vi "maximini_XYlist_svi.vi"(9 "stored XY":T1, 10 "LY":dbl, 11 "LX":dbl) -> (2 "mini (µm)":dbl, 3 "maxi (µm)":dbl)   [LabVIEW 2013]
uses:
  <vilib>/Analysis/Matrix/Datatypes/RealMatrix.ctl
  <vilib>/Analysis/Matrix/Numeric/Conversions/Matrix To Array - RM.vi
  <vilib>/Analysis/Matrix/NI_Matrix.lvlib
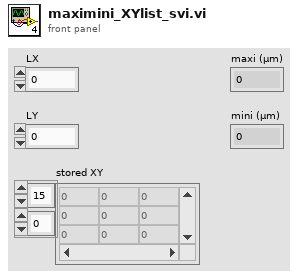
[diagram p1: front panel]
types:
  T1 = typedef "NI_Matrix.lvlib/RealMatrix.ctl" = dbl[][]
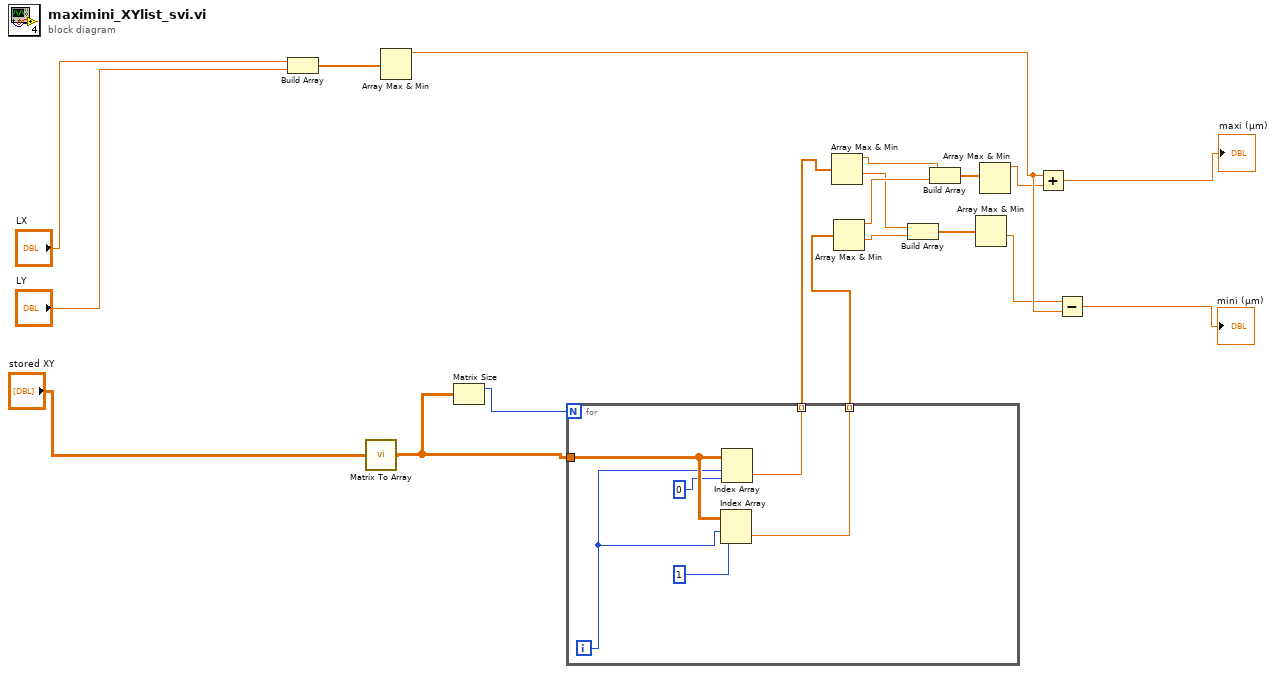
[diagram p0: block diagram]
diagram:
  n1 = Build Array("LX", "LY") -> (w8:dbl[])
  n2 = call-poly <vilib>:"Matrix To Array.vi"("Real Matrix"="stored XY") -> ("Real 2D Array"=w12:dbl[][])
  n3 = Array Max & Min(array=w8) -> (max value=w11:dbl)  [unwired: 3 out]
  n4 = Matrix Size(0:w12) -> (1:w1:i32)  [unwired: 1 out]
  n5 = for {
    N: w1 -> [_]
    tunnel: w12 -> [w25]
    tunnel: [w20] -> w13 mode=indexing
    tunnel: [w21] -> w14 mode=indexing
    i -> [w23]
    n6 = Index Array(array=w25, index (row)=w23, index (col)=1) -> (element=w21:dbl)
    n7 = Index Array(array=w25, index (row)=w23, index (col)=0) -> (element=w20:dbl)
  }
  n8 = Array Max & Min(array=w13) -> (max value=w2:dbl, min value=w4:dbl)  [unwired: 2 out]
  n9 = Array Max & Min(array=w14) -> (max value=w7:dbl, min value=w3:dbl)  [unwired: 2 out]
  n10 = Build Array(w4, w3) -> (w6:dbl[])
  n11 = Build Array(w2, w7) -> (w5:dbl[])
  n12 = Array Max & Min(array=w6) -> (min value=w9:dbl)  [unwired: 3 out]
  n13 = Array Max & Min(array=w5) -> (max value=w10:dbl)  [unwired: 3 out]
  n14 = Add(x=w11, y=w10) -> (x+y=→"maxi (µm)":dbl)
  n15 = Subtract(x=w9, y=w11) -> (x-y=→"mini (µm)":dbl)
